vi "Centrialize Error Handling.vi"(8 "error in (no error)":errorcluster, 9 "Error":errorcluster, 10 "Error Level":T1, 11 "Car Wash Controller Actor in":refnum<class "Car Wash Controller Actor.lvclass">) -> (0 "error out":errorcluster, 3 "Car Wash Controller Actor out":refnum<class "Car Wash Controller Actor.lvclass">)   [LabVIEW 2019, in "Car Wash Controller Actor.lvlib" / "Car Wash Controller Actor.lvclass"]
uses:
  Car Wash Controller Actor.lvclass
  <vilib>/ActorFramework/Actor/Actor.lvclass
  Car Wash Controller Actor Messages/Set State Msg/Set State Msg.lvclass
  State -Enum.ctl
  Error Levels.ctl
  C:/Program Files (x86)/National Instruments/LabVIEW 2019/vi.lib/ActorFramework/Actor/Actor.lvclass
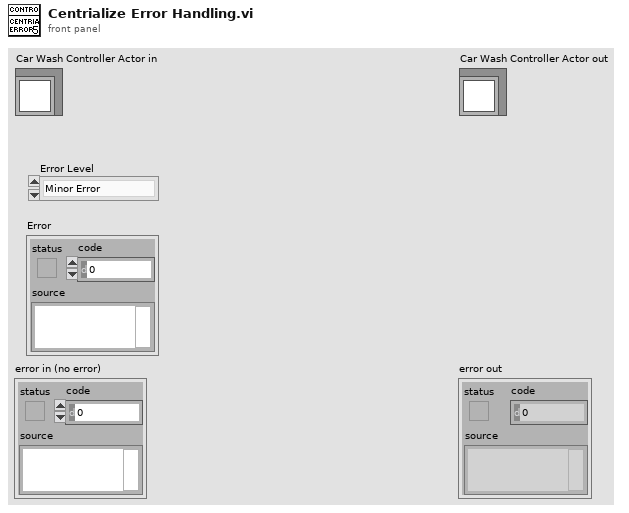
[diagram p1: front panel]
types:
  T1 = typedef "Car Wash Controller Actor.lvlib/Car Wash Controller Actor.lvclass/Error Levels.ctl" = enum16{"Minor Error", "Wash Cycle Error", "System Error"}
  T2 = cluster{"Description":string, "Error Level":T1, "Time and Date":timestamp, "Station":u32, "Step":string}
  T3 = typedef "Car Wash Controller Actor.lvlib/Car Wash Controller Actor.lvclass/State -Enum.ctl" = enum16{"Initial", "Wait for Start", "Start", "Wait for Vehicle Position", "Wash Step Execution", "Wash Step/Cycle Completion", "Wash Exit", "Wash Abort/Terminate"}
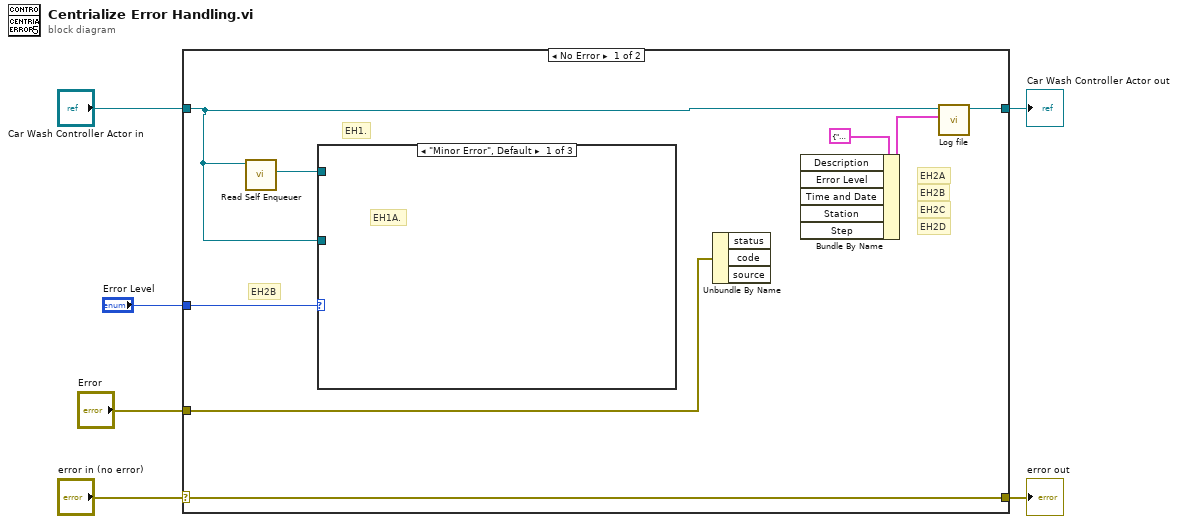
[diagram p0: block diagram]
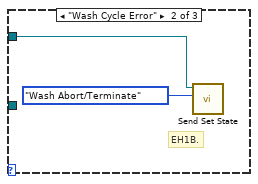
[diagram p2: hidden frame]
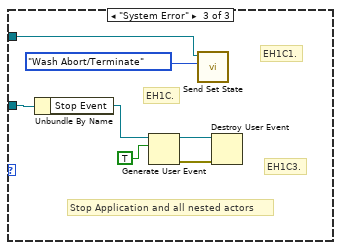
[diagram p3: hidden frame]
diagram:
  n1 = case shown="No Error" "error in (no error)" {
    selector: "error in (no error)" -> [w14 w25]
    tunnel: [w14 w25] -> w5
    tunnel: [w10 w24] -> w3
    tunnel: "Car Wash Controller Actor in" -> [w11 w24]
    tunnel: "Error Level" -> [w13 _]
    tunnel: "Error" -> [w7 _]
    frame No Error {
      # "EH2A"
      # "EH2D"
      # "EH2B"
      # "EH2C"
      # "EH1."
      # "EH2B"
      n2 = call <vilib>:"Read Self Enqueuer.vi"("Actor"=w11) -> ("Self Enqueuer"=w12:refnum<class "Message Enqueuer.lvclass">)  [unwired: 10 in]
      n3 = case shown="\"Minor Error\", Default" w13 {
        tunnel: w12 -> [_ w15 w23]
        tunnel: w11 -> [_ _ w21]
        frame "Minor Error", Default {
          # "EH1A."
        }
        frame "Wash Cycle Error" {
          # "EH1B."
          n4 = call "Send Set State.vi"("States"=State_-Enum."Wash Abort/Terminate", "Message Enqueuer"=w15) -> ()  [unwired: 8 in, 2 out]
        }
        frame "System Error" {
          # "EH1C1."
          # "Stop Application and all nested actors"
          # "EH1C3."
          # "EH1C."
          n5 = Unbundle By Name(w21) -> ("Stop Event"=w20:refnum<user-event>)
          n6 = Generate User Event(user event=w20, event data cluster=TRUE ("event data")) -> (user event out=w17:refnum<user-event>, error out=w18:errorcluster)  [unwired: 2 in]
          n7 = call "Send Set State.vi"("States"=State_-Enum."Wash Abort/Terminate", "Message Enqueuer"=w23) -> ()  [unwired: 8 in, 2 out]
          n8 = Destroy User Event(user event=w17, error in=w18) -> ()  [unwired: 1 out]
        }
      }
      n9 = Unbundle By Name(w7) -> ()  [unwired: 3 out]
      n10 = Bundle By Name(cluster=T2 {"Description"="", "Error Level"=enum."Minor Error", "Time and Date"=timestamp(0 s since 1904-01-01), "Station"=0, "Step"=""} ("Logging Data")) -> (w8:T2)  [unwired: 5 in]
      n11 = call "Log file.vi"("Logging Data"=w8, "Car Wash Controller Actor in"=w11) -> ("Car Wash Controller Actor out"=w10:refnum<class "Car Wash Controller Actor.lvclass">)  [unwired: 8 in, 1 out]
    }
    frame Error {
    }
  }
  "error out" <- w5
  "Car Wash Controller Actor out" <- w3
